vi "Top Level VI.vi"() -> ()   [LabVIEW 2020]
uses:
  builds/Project A/PPL/Library A.lvlibp
panel:
  out "String":string
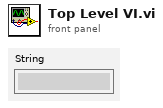
[diagram p1: front panel]
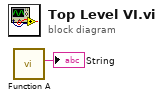
[diagram p0: block diagram]
diagram:
  n1 = call "Function A.vi"() -> ("String"=→"String":string)  [unwired: 11 in]
